vi "TalkToMCP.vi"   [LabVIEW 2011]
uses:
  Globals/CTCGlbs.vi
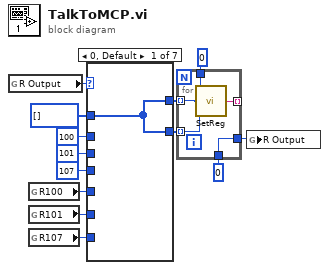
[diagram p0: block diagram]
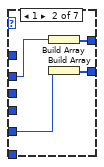
[diagram p2: hidden frame]
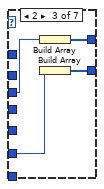
[diagram p3: hidden frame]
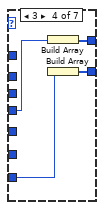
[diagram p4: hidden frame]
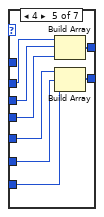
[diagram p5: hidden frame]
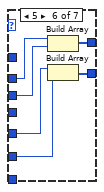
[diagram p6: hidden frame]
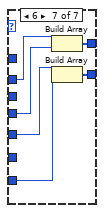
[diagram p7: hidden frame]
diagram:
  n1 = global read "CTCGlbs.vi" "R Output"() -> (w13:i32)
  n2 = global read "CTCGlbs.vi" "R100"() -> (w8:i32)
  n3 = global read "CTCGlbs.vi" "R101"() -> (w7:i32)
  n4 = global read "CTCGlbs.vi" "R107"() -> (w6:i32)
  n5 = case shown="0, Default" w13 {
    tunnel: i32[] [] -> [w14 _ _ _ _ _ _]
    tunnel: [w14 w17 w21 w25 w31 w38 w44] -> w5
    tunnel: [w14 w15 w19 w23 w27 w35 w41] -> w4
    tunnel: u16 100 ("Register Number") -> [_ w18 _ _ w34 w40 w46]
    tunnel: u16 101 -> [_ _ w22 _ w33 w39 _]
    tunnel: u16 107 -> [_ _ _ w26 w32 _ w45]
    tunnel: w8 -> [_ w16 _ _ w30 w37 w43]
    tunnel: w7 -> [_ _ w20 _ w29 w36 _]
    tunnel: w6 -> [_ _ _ w24 w28 _ w42]
    frame 0, Default {
    }
    frame 1 {
      n6 = Build Array(w18) -> (w17:u16[])
      n7 = Build Array(w16) -> (w15:i32[])
    }
    frame 2 {
      n8 = Build Array(w22) -> (w21:u16[])
      n9 = Build Array(w20) -> (w19:i32[])
    }
    frame 3 {
      n10 = Build Array(w26) -> (w25:u16[])
      n11 = Build Array(w24) -> (w23:i32[])
    }
    frame 4 {
      n12 = Build Array(w34, w33, w32) -> (w31:u16[])
      n13 = Build Array(w30, w29, w28) -> (w27:i32[])
    }
    frame 5 {
      n14 = Build Array(w40, w39) -> (w38:u16[])
      n15 = Build Array(w37, w36) -> (w35:i32[])
    }
    frame 6 {
      n16 = Build Array(w46, w45) -> (w44:u16[])
      n17 = Build Array(w43, w42) -> (w41:i32[])
    }
  }
  n18 = for {
    tunnel: w5 -> [w51] mode=indexing
    tunnel: w4 -> [w50] mode=indexing
    tunnel: [w49] -> _ mode=indexing
    tunnel: [w48] -> w2
    tunnel: 0 -> [w48]
    tunnel: u32 0 ("Controller ID") -> [w47]
    n19 = call "SetReg.vi"("SetReg"=w50, "Register"=w51, "Controller ID"=w47) -> ("Err Msg"=w49:string)  [unwired: 1 out]
  }
  n20 = global write "CTCGlbs.vi" "R Output"(w2) -> ()
